vi "MAIN_TWO_PORTS.vi"(6 "ECU TYPE":u16(ring) items=["LSMD", "LSMP", "LSMRL", "LSMRR"]) -> (0 "Data By ID OK":bool, 1 "Hall Test 3 OK":bool, 2 "Sleep Request OK":bool, 3 "Hall Test 1 OK":bool, 4 "SBC OK":bool, 5 "Hall Test 2 OK":bool, 7 "Hard Reset OK":bool, 8 "BIST OK":bool, 9 "SW Version OK":bool, 10 "ECU ID OK":bool, 11 "Session OK":bool)   [LabVIEW 2023]
uses:
  Sub VIs/Global .vi
panel:
  out "ReplyTracMex":string
  out "Trazabilidad":bool
  in  "Trazabilidad\nOFF  /  ON":bool
  in  "Stop":bool
  in  "Start":bool
  out "Puerto DAQ":i32
  out "Respuesta Trazabilidad":string
  out "Finish Time":string
  out "Start Time":string
  out "Status":i8
  in  "Número Serial":string
  out "Enter Brose Ext OK":bool
  out "Hall Test 3 Response":string
  out "Enter Brose Ext":string
  out "ECU Hard Reset":string
  out "Program SBC":string
  out "ID Response":string
  out "ID Request":string
  out "Tester Present OK":bool
  out "Hall Test 2 Response":string
  out "Hall Test 1 Response":string
  out "Supply Voltage ADC Response":string
  out "Self Test BIST":string
  out "Sleep Request Response":string
  out "Read Data By ID":string
  out "Verify ECU ID String":string
  out "Verify SW Version":string
  out "Tester Present Command":string
  out "Enter Brose EOL Ext Session":string
  # "*Revisar debido a cambio en respuesta"
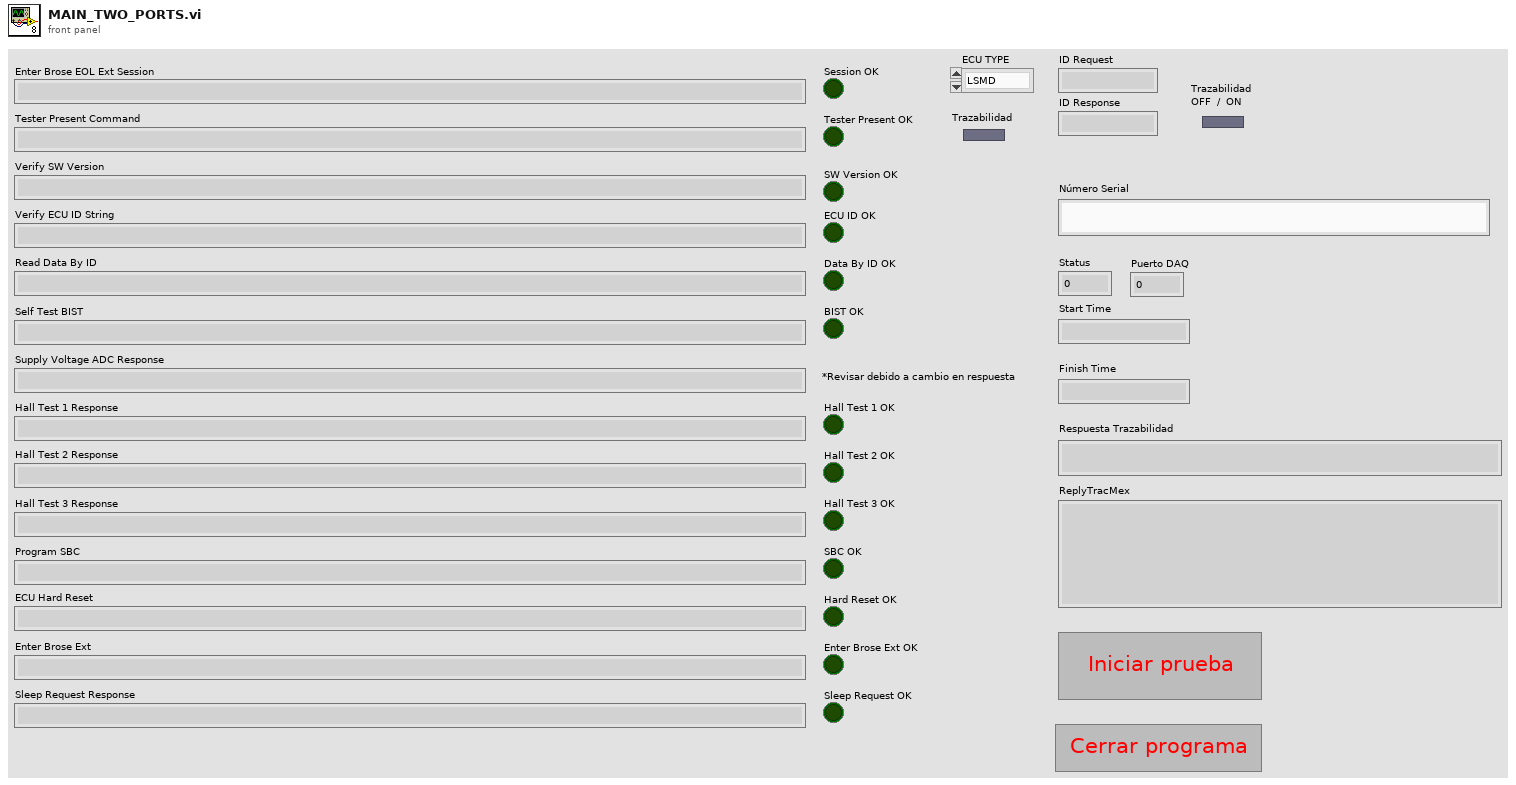
[diagram p1: front panel]
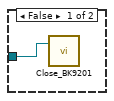
[diagram p2: hidden frame]
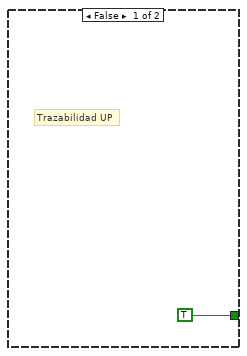
[diagram p3: hidden frame]
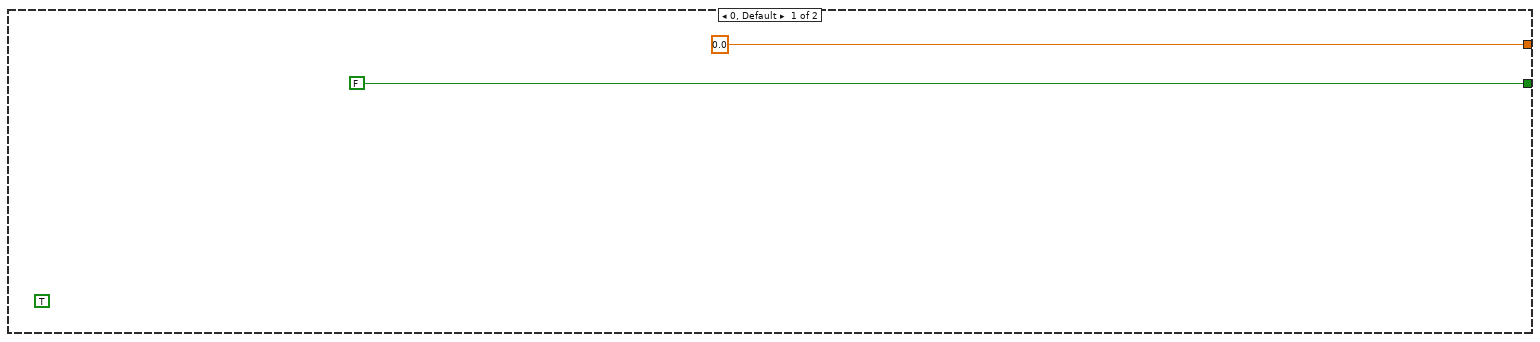
[diagram p4: hidden frame]
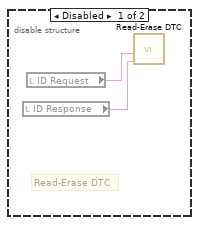
[diagram p5: hidden frame]
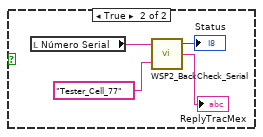
[diagram p6: hidden frame]
diagram:
  n1 = call "Initalization_BK9201.vi"("Instrument In"=refnum<visa-resource-name> "USB0::0x2EC7::0x9200::800889011776910056::INSTR") -> ("Instrument Out"=w1:refnum<visa-resource-name>)  [unwired: 3 in, 1 out]
  n2 = while {
    tunnel: w1 -> [w5]
    stop <- w4 stop-if-true
    n3 = while {
      tunnel: ["Stop"] -> w4
      tunnel: [w256] -> w3
      stop <- w261 stop-if-true
      n4 = Wait (ms)(milliseconds to wait=u32 100) -> ()  [unwired: 1 out]
      n5 = Select(t=FALSE, s="Stop", f=TRUE) -> (s? t:f=w256:bool)
      n6 = Or(x="Stop", y="Start") -> (x .or. y?=w261:bool)
      "Trazabilidad" <- "Trazabilidad\nOFF  /  ON"
    }
    n7 = case shown="True" w3 {
      tunnel: w5 -> [w6 w8]
      frame False {
        n8 = call "Close_BK9201.vi"("Instrument In"=w6) -> ()  [unwired: 2 in, 1 out]
      }
      frame True {
        n9 = flat-sequence {
          tunnel: w8 -> [w243]
          tunnel: [w245] -> w9
          tunnel: [w254] -> w7
          frame #0 {
            n10 = call "Display Message to User"("Message"="COLOCA LA PIEZA EN EL NIDO.\n\nCIERRA EL NIDO Y PRESIONA OK.") -> ()  [unwired: 9 in, 2 out]
          }
          frame #1 {
            w244 = u16 1 items=["Disable", "Enable"] ("Ring")
            n11 = call "Setting_BK9201.vi"("Instrument In"=w243, "Set Out Voltage"=9.0, "Current Limit"=1.0, "Ring"=w244) -> ("Instrument Out"=w245:refnum<visa-resource-name>)  [unwired: 14 in, 1 out]
          }
          frame #2 {
            n12 = local read "Trazabilidad"() -> (w248:bool)
            n13 = case shown="False" w248 {
              frame False {
                n14 = local write "Status"(i8 1 ("Status 2")) -> ()
              }
              frame True {
                n15 = local read "Número Serial"() -> (w252:string)
                n16 = call "WSP2_BackCheck_Serial.vi"("serialNumber"=w252, "stationName"="Tester_Cell_77") -> ("Status"=→"Status":i8, "ReplyTracMex"=→"ReplyTracMex":string)  [unwired: 1 out]
              }
            }
          }
          frame #3 {
            n17 = local read "Status"() -> (w254:i8)
          }
        }
        n18 = case shown="1" w7 {
          tunnel: [FALSE w24] -> w12
          tunnel: [0.0 ("f") w31] -> w11
          tunnel: w9 -> [_ w26]
          frame 0, Default {
            (unwired) TRUE
          }
          frame 1 {
            n19 = flat-sequence {
              tunnel: [w80] -> w67
              tunnel: [w79] -> w66
              tunnel: w67 -> [w88]
              tunnel: w66 -> [w87]
              tunnel: [w86] -> w65
              tunnel: [w85] -> w64
              tunnel: [w93] -> w63
              tunnel: [w94] -> w62
              tunnel: w65 -> [w96]
              tunnel: w64 -> [w95]
              tunnel: [w101] -> w61
              tunnel: [w102] -> w60
              tunnel: w63 -> [w104]
              tunnel: w62 -> [w103]
              tunnel: [w110] -> w58
              tunnel: [w109] -> w59
              tunnel: w61 -> [w112]
              tunnel: w60 -> [w111]
              tunnel: [w116] -> w57
              tunnel: [w115] -> w56
              tunnel: w59 -> [w117]
              tunnel: w58 -> [w118]
              tunnel: [w127] -> w28
              tunnel: [w126] -> w30
              tunnel: w57 -> [w122]
              tunnel: w56 -> [w121]
              tunnel: w30 -> [w134]
              tunnel: [w134] -> w29
              tunnel: w28 -> [w133]
              tunnel: [w133] -> w27
              tunnel: w26 -> [w129]
              tunnel: [w128] -> w25
              tunnel: w29 -> [w138]
              tunnel: w27 -> [w137]
              tunnel: [w136] -> w55
              tunnel: [w135] -> w54
              tunnel: [w148] -> w53
              tunnel: [w147] -> w52
              tunnel: w55 -> [w142]
              tunnel: w54 -> [w141]
              tunnel: w53 -> [w152]
              tunnel: w52 -> [w151]
              tunnel: [w150] -> w51
              tunnel: [w149] -> w50
              tunnel: [w162] -> w49
              tunnel: [w161] -> w48
              tunnel: w51 -> [w156]
              tunnel: w50 -> [w155]
              tunnel: w49 -> [w165]
              tunnel: w48 -> [w166]
              tunnel: [w164] -> w47
              tunnel: [w163] -> w46
              tunnel: [w176] -> w45
              tunnel: [w175] -> w44
              tunnel: w47 -> [w170]
              tunnel: w46 -> [w169]
              tunnel: [w178] -> w43
              tunnel: w45 -> [w178]
              tunnel: [w177] -> w42
              tunnel: w44 -> [w177]
              tunnel: [w186] -> w41
              tunnel: [w185] -> w40
              tunnel: w43 -> [w184]
              tunnel: w42 -> [w183]
              tunnel: w41 -> [w194]
              tunnel: w40 -> [w193]
              tunnel: [w192] -> w39
              tunnel: [w191] -> w38
              tunnel: w39 -> [w199]
              tunnel: [w199] -> w37
              tunnel: w38 -> [w198]
              tunnel: [w198] -> w36
              tunnel: w37 -> [w207]
              tunnel: w36 -> [w206]
              tunnel: [w203] -> w35
              tunnel: [w202] -> w34
              tunnel: [w213] -> w32
              tunnel: [w212] -> w33
              tunnel: w35 -> [w211]
              tunnel: w34 -> [w210]
              tunnel: w33 -> [w216]
              tunnel: w32 -> [w217]
              tunnel: w25 -> [w218]
              tunnel: [w231] -> w31
              tunnel: [w228] -> w24
              frame #0 {
                w69 = FALSE
                w68 = ""
                n20 = local write "Hard Reset OK"(w69) -> ()
                n21 = local write "Sleep Request OK"(w69) -> ()
                n22 = local write "Enter Brose Ext OK"(w69) -> ()
                n23 = local write "SBC OK"(w69) -> ()
                n24 = local write "ECU ID OK"(w69) -> ()
                n25 = local write "Data By ID OK"(w69) -> ()
                n26 = local write "SW Version OK"(w69) -> ()
                n27 = local write "Tester Present OK"(w69) -> ()
                n28 = local write "Session OK"(w69) -> ()
                n29 = local write "Hall Test 2 OK"(w69) -> ()
                n30 = local write "Hall Test 3 OK"(w69) -> ()
                n31 = local write "BIST OK"(w69) -> ()
                n32 = local write "Hall Test 1 OK"(w69) -> ()
                n33 = local write "Enter Brose EOL Ext Session"(w68) -> ()
                n34 = local write "Supply Voltage ADC Response"(w68) -> ()
                n35 = local write "Tester Present Command"(w68) -> ()
                n36 = local write "Sleep Request Response"(w68) -> ()
                n37 = local write "Enter Brose Ext"(w68) -> ()
                n38 = local write "Finish Time"(w68) -> ()
                n39 = local write "ECU Hard Reset"(w68) -> ()
                n40 = local write "Respuesta Trazabilidad"(w68) -> ()
                n41 = local write "Hall Test 1 Response"(w68) -> ()
                n42 = local write "ReplyTracMex"(w68) -> ()
                n43 = local write "Hall Test 3 Response"(w68) -> ()
                n44 = local write "Verify ECU ID String"(w68) -> ()
                n45 = local write "Program SBC"(w68) -> ()
                n46 = local write "Hall Test 2 Response"(w68) -> ()
                n47 = local write "Verify SW Version"(w68) -> ()
                n48 = local write "Start Time"(w68) -> ()
                n49 = local write "Read Data By ID"(w68) -> ()
                n50 = local write "Self Test BIST"(w68) -> ()
              }
              frame #1 {
                n51 = call "WSP2_GetDateTimeStr.vi"() -> ("Time"=→"Start Time":string)  [unwired: 1 in, 1 out]
              }
              frame #2 {
                # "ECU SELECT"
                n52 = global write "Global .vi" "ECU TYPE"("ECU TYPE") -> ()
                n53 = call "ECU Selector.vi"("ECU TYPE"="ECU TYPE") -> ("ID Response"=→"ID Response":string, "Puerto DAQ"=→"Puerto DAQ":i32, "ID Request"=→"ID Request":string)  [unwired: 1 in, 2 out]
              }
              frame #3 {
                # "Comunication Startup"
                n54 = local read "ID Request"() -> (w77:string)
                n55 = local read "ID Response"() -> (w76:string)
                n56 = call "Session Request - Brose Session.vi"("ID Request"=w77, "ID Response"=w76) -> ("Data String"=w78:string, "Write"=w80:refnum<k21>, "Read"=w79:refnum<k21>)  [unwired: 1 out]
                "Enter Brose EOL Ext Session" <- w78
                n57 = call "Evaluate Session.vi"("String In"=w78) -> ("Test OK"=→"Session OK":bool)
              }
              frame #4 {
                # "Tester Present Command"
                n58 = local read "ID Response"() -> (w81:string)
                n59 = local read "ID Request"() -> (w82:string)
                n60 = call "Tester Present Command.vi"("ID Response"=w81, "ID Request"=w82, "Read"=w87, "Write"=w88) -> ("Read out"=w86:refnum<k21>, "Write out"=w85:refnum<k21>, "Data String 2"=w84:string)  [unwired: 1 out]
                "Tester Present Command" <- w84
                n61 = call "Evaluate Tester Present.vi"("String In"=w84) -> ("Test OK"=→"Tester Present OK":bool)
              }
              frame #5 {
                # "Verify SW Version"
                n62 = local read "ID Response"() -> (w89:string)
                n63 = local read "ID Request"() -> (w90:string)
                n64 = call "Verify SW Version.vi"("ID Response"=w89, "ID Request"=w90, "Read"=w96, "Write"=w95) -> ("Data String 3"=w92:string, "Write out"=w94:refnum<k21>, "Read out"=w93:refnum<k21>)  [unwired: 1 out]
                "Verify SW Version" <- w92
                n65 = call "Evaluate SW Version Response.vi"("String In"=w92) -> ("Test OK"=→"SW Version OK":bool)
              }
              frame #6 {
                # "Verify ECU ID String"
                n66 = local read "ID Response"() -> (w99:string)
                n67 = local read "ID Request"() -> (w100:string)
                n68 = call "Verify ECU ID String.vi"("ID Response"=w99, "ID Request"=w100, "Read"=w104, "Write"=w103) -> ("Data String 3"=w98:string, "Write out"=w102:refnum<k21>, "Read out"=w101:refnum<k21>)  [unwired: 1 out]
                "Verify ECU ID String" <- w98
                n69 = call "Evaluate ECU ID String.vi"("String In"=w98) -> ("Test OK"=→"ECU ID OK":bool)
              }
              frame #7 {
                # "Start Routine Read Data By ID"
                n70 = local read "ID Response"() -> (w107:string)
                n71 = local read "ID Request"() -> (w108:string)
                n72 = call "Start Routine - Read Data ID.vi"("ID Response"=w107, "ID Request"=w108, "Read"=w112, "Write"=w111) -> ("Data String 3"=w106:string, "Write out"=w110:refnum<k21>, "Read out"=w109:refnum<k21>)  [unwired: 1 out]
                "Read Data By ID" <- w106
                n73 = call "Evaluate Read Data By ID.vi"("String In"=w106) -> ("Test OK"=→"Data By ID OK":bool)
              }
              frame #8 {
                # "Selt Test BIST"
                n74 = local read "ID Response"() -> (w119:string)
                n75 = local read "ID Request"() -> (w120:string)
                n76 = call "Self Test BIST.vi"("ID Response"=w119, "ID Request"=w120, "Read"=w117, "Write"=w118) -> ("Data String 3"=w113:string, "Write out"=w115:refnum<k21>, "Read out"=w116:refnum<k21>)  [unwired: 1 out]
                "Self Test BIST" <- w113
                n77 = call "Evaluate Self Test BIST.vi"("String In"=w113) -> ("Test OK"=→"BIST OK":bool)
              }
              frame #9 {
                # "Supply Voltage ADC Measurement"
                n78 = local read "ID Response"() -> (w123:string)
                n79 = local read "ID Request"() -> (w124:string)
                n80 = call "Supply Voltage ADC Measurement.vi"("ID Response"=w123, "ID Request"=w124, "Read"=w122, "Write"=w121) -> ("Data String 3"=→"Supply Voltage ADC Response":string, "Write out"=w127:refnum<k21>, "Read out"=w126:refnum<k21>)  [unwired: 1 out]
              }
              frame #10 {
                w130 = u16 1 items=["Disable", "Enable"] ("Ring")
                n81 = call "Setting_BK9201.vi"("Instrument In"=w129, "Set Out Voltage"=12.0, "Current Limit"=1.0, "Ring"=w130) -> ("Instrument Out"=w128:refnum<visa-resource-name>)  [unwired: 14 in, 1 out]
              }
              frame #11 {
                # "Display Message I"
                n82 = global read "Global .vi" "ECU TYPE"() -> (w140:u16)
                n83 = call "Cuadro de Texto.vi"("Numeric"=1.0, "Read"=w138, "Write"=w137, "ECU TYPE"=w140) -> ("Write out"=w135:refnum<k21>, "Read out"=w136:refnum<k21>)
              }
              frame #12 {
                # "Hall Test 1"
                n84 = local read "ID Response"() -> (w145:string)
                n85 = local read "ID Request"() -> (w146:string)
                n86 = call "Hall Test.vi"("ID Response"=w145, "ID Request"=w146, "Read"=w142, "Write"=w141) -> ("Data String 3"=w144:string, "Write out"=w147:refnum<k21>, "Read out"=w148:refnum<k21>)  [unwired: 1 out]
                "Hall Test 1 Response" <- w144
                n87 = call "Evaluate Hall Test 1.vi"("String In"=w144) -> ("Test OK"=→"Hall Test 1 OK":bool)
              }
              frame #13 {
                # "Display Message II"
                n88 = global read "Global .vi" "ECU TYPE"() -> (w154:u16)
                n89 = call "Cuadro de Texto.vi"("Numeric"=2.0, "Read"=w152, "Write"=w151, "ECU TYPE"=w154) -> ("Write out"=w149:refnum<k21>, "Read out"=w150:refnum<k21>)
              }
              frame #14 {
                # "Hall Test 2"
                n90 = local read "ID Response"() -> (w159:string)
                n91 = local read "ID Request"() -> (w160:string)
                n92 = call "Hall Test.vi"("ID Response"=w159, "ID Request"=w160, "Read"=w156, "Write"=w155) -> ("Data String 3"=w158:string, "Write out"=w162:refnum<k21>, "Read out"=w161:refnum<k21>)  [unwired: 1 out]
                "Hall Test 2 Response" <- w158
                n93 = call "Evaluate Hall Test 2.vi"("String In"=w158) -> ("Test OK"=→"Hall Test 2 OK":bool)
              }
              frame #15 {
                # "Display Mesagge III"
                n94 = global read "Global .vi" "ECU TYPE"() -> (w168:u16)
                n95 = call "Cuadro de Texto.vi"("Numeric"=3.0, "Read"=w166, "Write"=w165, "ECU TYPE"=w168) -> ("Write out"=w163:refnum<k21>, "Read out"=w164:refnum<k21>)
              }
              frame #16 {
                # "Hall Test 3"
                n96 = local read "ID Request"() -> (w174:string)
                n97 = local read "ID Response"() -> (w173:string)
                n98 = call "Hall Test.vi"("ID Response"=w173, "ID Request"=w174, "Read"=w170, "Write"=w169) -> ("Data String 3"=w172:string, "Write out"=w175:refnum<k21>, "Read out"=w176:refnum<k21>)  [unwired: 1 out]
                "Hall Test 3 Response" <- w172
                n99 = call "Evaluate Hall Test 3.vi"("String In"=w172) -> ("Test OK"=→"Hall Test 3 OK":bool)
              }
              frame #17 {
                n100 = disable-structure shown="Enabled" {
                  frame Disabled {
                    # "Read-Erase DTC"
                    n101 = local read "ID Response"() -> (w179:string)
                    n102 = local read "ID Request"() -> (w180:string)
                    n103 = call "Read-Erase DTC.vi"("ID Response"=w179, "ID Request"=w180) -> ()  [unwired: 2 in, 4 out]
                  }
                  frame Enabled {
                  }
                }
              }
              frame #18 {
                # "Program SBC"
                n104 = local read "ID Response"() -> (w187:string)
                n105 = local read "ID Request"() -> (w188:string)
                n106 = call "Routine Before BIST.vi"("ID Response"=w187, "ID Request"=w188, "Read"=w184, "Write"=w183) -> ("Data String 3"=w182:string, "Write out"=w185:refnum<k21>, "Read out"=w186:refnum<k21>)  [unwired: 1 out]
                "Program SBC" <- w182
                n107 = call "Evaluate SBC.vi"("String In"=w182) -> ("Test OK"=→"SBC OK":bool)
              }
              frame #19 {
                # "ECU Hard Reset"
                n108 = local read "ID Request"() -> (w195:string)
                n109 = local read "ID Response"() -> (w196:string)
                n110 = call "Routine Before BIST I.vi"("ID Response"=w196, "ID Request"=w195, "Read"=w194, "Write"=w193) -> ("Data String 3"=w190:string, "Write out"=w192:refnum<k21>, "Read out"=w191:refnum<k21>)  [unwired: 1 out]
                "ECU Hard Reset" <- w190
                n111 = call "Evaluate ECU Hard Reset.vi"("String In"=w190) -> ("Test OK"=→"Hard Reset OK":bool)
              }
              frame #20 {
                n112 = Wait (ms)(milliseconds to wait=u32 250) -> ()  [unwired: 1 out]
              }
              frame #21 {
                n113 = local read "ID Request"() -> (w205:string)
                n114 = local read "ID Response"() -> (w204:string)
                n115 = call "Session Request II.vi"("ID Response"=w204, "ID Request"=w205, "Read"=w206, "Write"=w207) -> ("Data String 3"=w201:string, "Write out"=w203:refnum<k21>, "Read out"=w202:refnum<k21>)  [unwired: 1 out]
                "Enter Brose Ext" <- w201
                n116 = call "Evaluate Session.vi"("String In"=w201) -> ("Test OK"=→"Enter Brose Ext OK":bool)
              }
              frame #22 {
                # "Sleep Current Measurement"
                n117 = local read "ID Request"() -> (w215:string)
                n118 = local read "ID Response"() -> (w214:string)
                n119 = call "Sleep Request.vi"("ID Response"=w214, "ID Resquest"=w215, "Read"=w210, "Write"=w211) -> ("Data String 3"=w209:string, "Write out"=w212:refnum<k21>, "Read out"=w213:refnum<k21>)  [unwired: 1 out]
                "Sleep Request Response" <- w209
                n120 = call "Evaluate Sleep Request.vi"("String In"=w209) -> ("Test OK"=→"Sleep Request OK":bool)
              }
              frame #23 {
                # "Cierra y\nlimpia puerto\nCAN"
                n121 = call <vilib>:"XNET Clear.vi"("session in"=w217) -> ()  [unwired: 14 in, 1 out]
                n122 = call <vilib>:"XNET Clear.vi"("session in"=w216) -> ()  [unwired: 14 in, 1 out]
              }
              frame #24 {
                w220 = u16 0 items=["Disable", "Enable"] ("Ring")
                # "Desactiva fuente"
                n123 = call "Setting_BK9201.vi"("Instrument In"=w218, "Set Out Voltage"=0.0, "Ring"=w220) -> ()  [unwired: 15 in, 2 out]
              }
              frame #25 {
                # "Descarga de capacitor"
                n124 = flat-sequence {
                  tunnel: w222 -> [w223]
                  tunnel: [w223] -> w221
                  tunnel: w221 -> [w225]
                  frame #0 {
                    n125 = call "DAQ Activate Output LINE 0.vi"("Puerto"=w223, "data"=TRUE) -> ()  [unwired: 4 in, 2 out]
                  }
                  frame #1 {
                    n126 = call "DAQ Desactivate Output LINE 0.vi"("Puerto"=w225, "data"=FALSE) -> ()  [unwired: 4 in, 2 out]
                  }
                }
                n127 = local read "Puerto DAQ"() -> (w222:i32)
              }
              frame #26 {
                # "Recibe tiempo final de prueba"
                n128 = call "WSP2_GetDateTimeStr.vi"() -> ("Time"=→"Finish Time":string)  [unwired: 1 in, 1 out]
              }
              frame #27 {
                # "Revivisa que haya pasado las pruebas"
                n129 = local read "Data By ID OK"() -> (w236:bool)
                n130 = local read "ECU ID OK"() -> (w237:bool)
                n131 = local read "Sleep Request OK"() -> (w229:bool)
                n132 = local read "SW Version OK"() -> (w238:bool)
                n133 = local read "BIST OK"() -> (w235:bool)
                n134 = local read "Session OK"() -> (w239:bool)
                n135 = local read "SBC OK"() -> (w230:bool)
                n136 = Compound Arithmetic op=AND(w239, w238, w237, w236, w235, w230, w229) -> (w234:bool)
                n137 = Select(t=1.0, s=w234, f=0.0) -> (s? t:f=w231:dbl)
                n138 = local read "Trazabilidad"() -> (w228:bool)
              }
            }
          }
        }
        n139 = case shown="True" w12 {
          tunnel: w11 -> [_ w17]
          tunnel: [TRUE TRUE] -> w10
          frame False {
            # "Trazabilidad UP"
          }
          frame True {
            # "Trazabilidad UP"
            n140 = local read "Número Serial"() -> (w21:string)
            n141 = local read "Start Time"() -> (w19:string)
            n142 = local read "Finish Time"() -> (w18:string)
            n143 = call "WSP2_InsertProcessDataWithFails.vi"("EndTime"=w18, "EntryTime"=w19, "PassFail"=w17, "ProcessName"="FUNCIONAL TEST > TOP", "StationName"="Tester_Cell_77", "SerialNumber"=w21) -> ("ReplyTrace"=→"Respuesta Trazabilidad":string)  [unwired: 4 in, 1 out]
          }
        }
        n144 = flat-sequence {
          tunnel: w10 -> [w240]
          frame #0 {
            # "Mensaje de retirar pieza"
            n145 = call "Display Message to User2"("Enable"=w240, "Message"="RETIRE LA PIEZA DEL NIDO") -> ()  [unwired: 8 in, 2 out]
          }
        }
      }
    }
  }
